vi "Cuboid collision and min distance test.vi"(2 "Cuboid 2":T1={"Vertices (x, y)"=[[0.0, 0.0], [0.0, 0.0], [0.0, 0.0], [0.0, 0.0]], "Zmin"=0.0, "Zmax"=0.0, "Centroid (x, y)"=[0.0, 0.0], "Radius"=0.0, "Edge normals (x, y)"=[[0.0, 0.0], [0.0, 0.0], [0.0, 0.0], [0.0, 0.0]], "Edge vectors (x, y)"=[[0.0, 0.0], [0.0, 0.0], [0.0, 0.0], [0.0, 0.0]]}, 3 "Cuboid 1":T1={"Vertices (x, y)"=[[0.0, 0.0], [0.0, 0.0], [0.0, 0.0], [0.0, 0.0]], "Zmin"=0.0, "Zmax"=0.0, "Centroid (x, y)"=[0.0, 0.0], "Radius"=0.0, "Edge normals (x, y)"=[[0.0, 0.0], [0.0, 0.0], [0.0, 0.0], [0.0, 0.0]], "Edge vectors (x, y)"=[[0.0, 0.0], [0.0, 0.0], [0.0, 0.0], [0.0, 0.0]]}) -> (0 "Minimum separation":dbl, 1 "Collision":bool)   [LabVIEW 2013]
uses:
  Cuboid properties.ctl
  <vilib>/Analysis/baseanly.llb/Real Dot Product.vi
  <vilib>/Analysis/NI_AALBase.lvlib
panel:
  # "PN 30/08/2014"
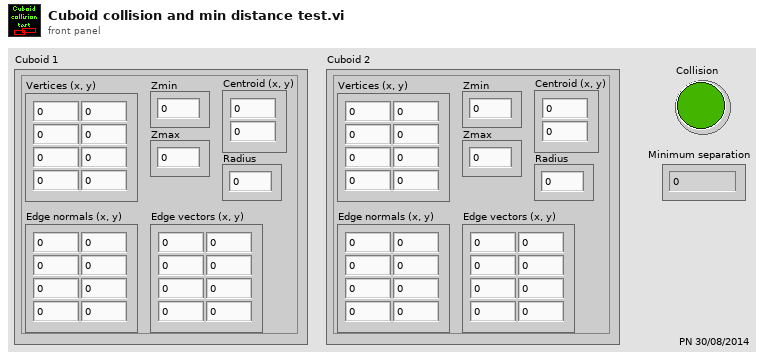
[diagram p1: front panel]
types:
  T1 = typedef "Cuboid properties.ctl" = cluster{"Vertices (x, y)":dbl[][], "Zmin":dbl, "Zmax":dbl, "Centroid (x, y)":dbl[], "Radius":dbl, "Edge normals (x, y)":dbl[][], "Edge vectors (x, y)":dbl[][]}
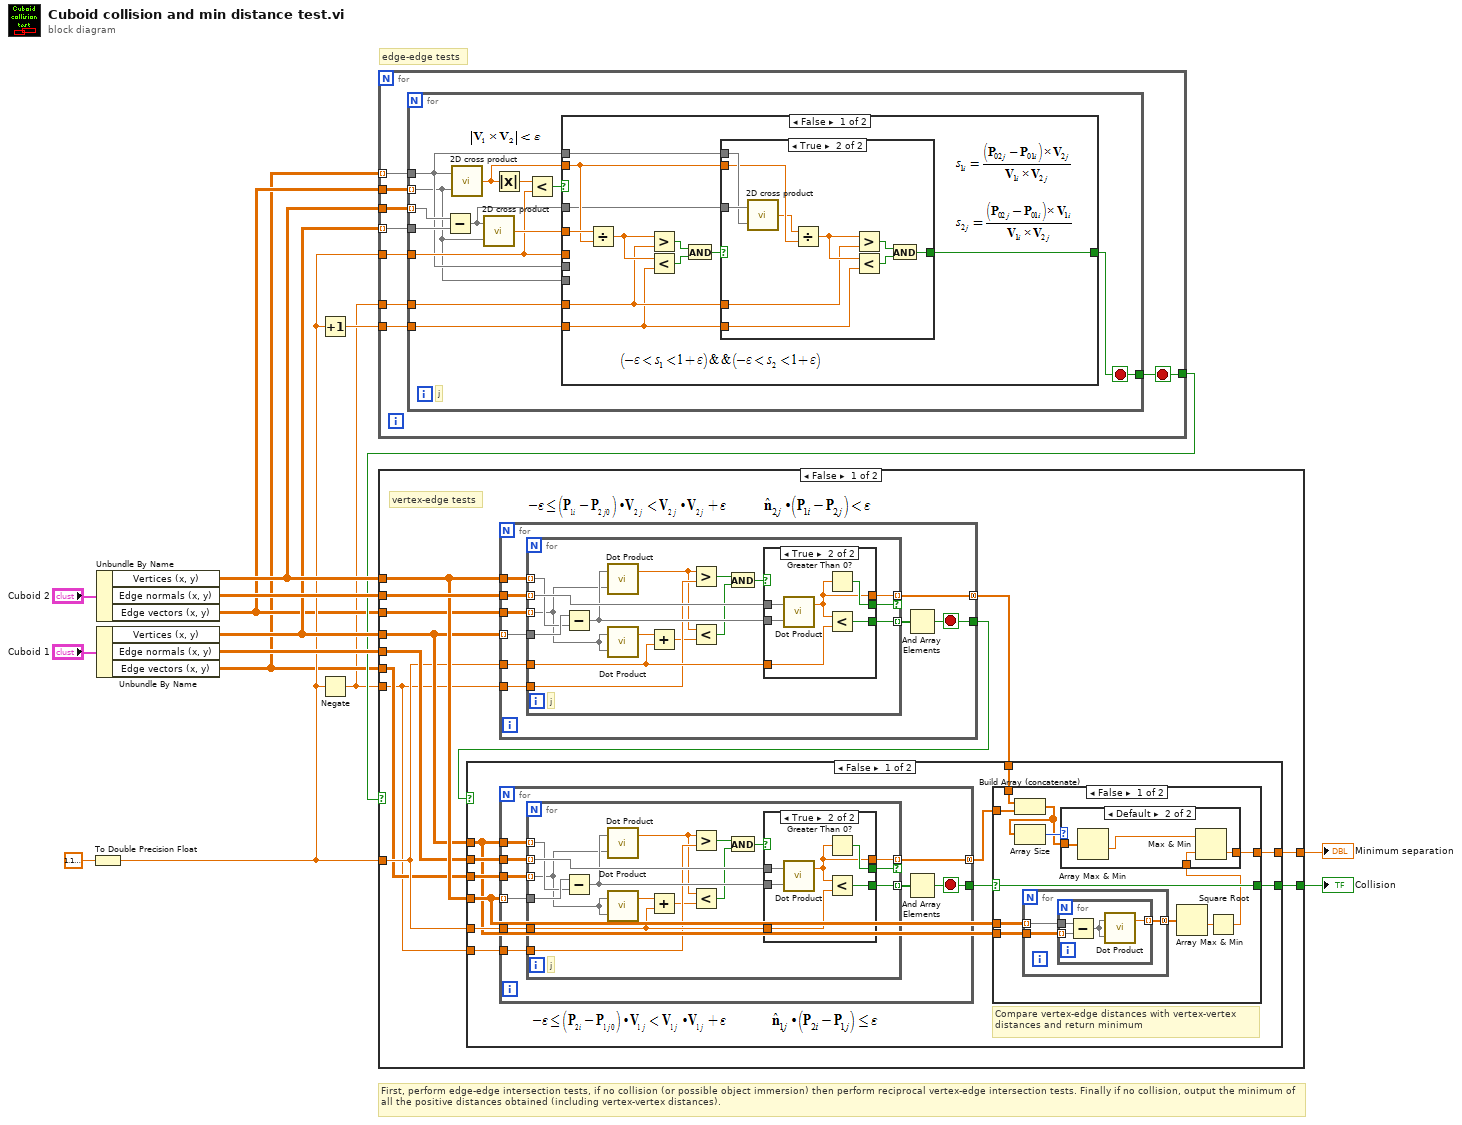
[diagram p0: block diagram]
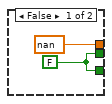
[diagram p2: hidden frame]
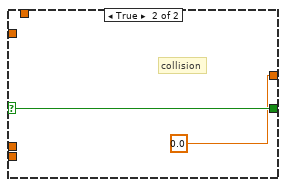
[diagram p4: hidden frame]
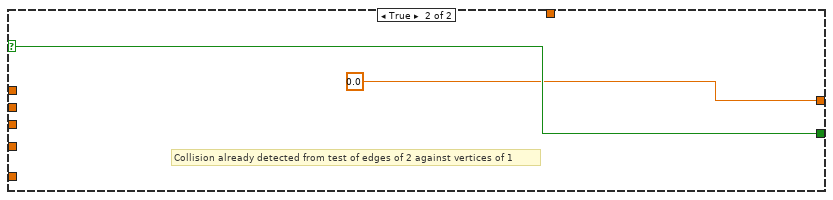
[diagram p5: hidden frame]
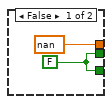
[diagram p6: hidden frame]
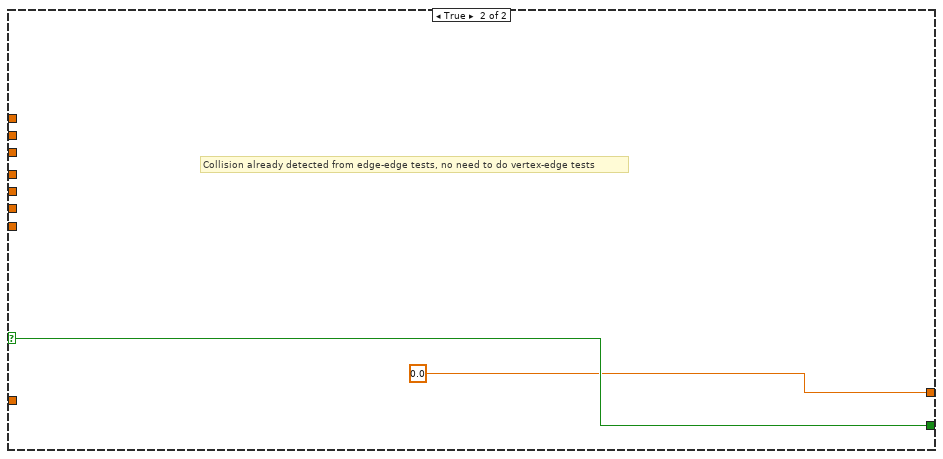
[diagram p7: hidden frame]
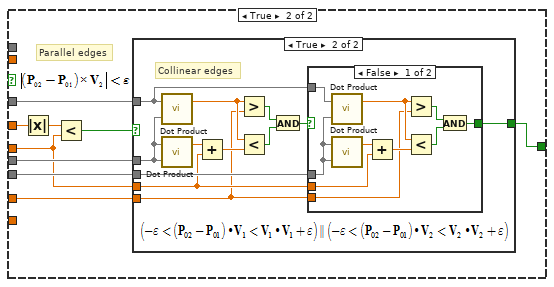
[diagram p9: hidden frame]
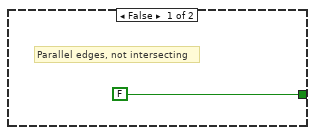
[diagram p10: hidden frame]
diagram:
  # "edge-edge tests"
  # "First, perform edge-edge intersection tests, if no collision (or possible object immersion) then perform reciprocal vertex-edge intersection tests. Finally if no collision, output the minimum of all the positive distances obtained (including vertex-vertex distances)."
  n1 = To Double Precision Float(number=sgl 1.1920929e-07) -> (double precision float=w5:dbl)
  n2 = Unbundle By Name("Cuboid 2") -> ("Vertices (x, y)"=w10:dbl[][], "Edge normals (x, y)"=w13:dbl[][], "Edge vectors (x, y)"=w3:dbl[][])
  n3 = Unbundle By Name("Cuboid 1") -> ("Vertices (x, y)"=w8:dbl[][], "Edge normals (x, y)"=w9:dbl[][], "Edge vectors (x, y)"=w2:dbl[][])
  n4 = Increment(x=w5) -> (x+1=w7:dbl)
  n5 = Negate(x=w5) -> (-x=w1:dbl)
  n6 = for {
    tunnel: w2 -> [w23] mode=indexing
    tunnel: w3 -> [w22]
    tunnel: w10 -> [w21]
    tunnel: w8 -> [w20] mode=indexing
    tunnel: w1 -> [w19]
    tunnel: w7 -> [w18]
    tunnel: w5 -> [w17]
    tunnel: [w16] -> w4
    stop <- w16 stop-if-true
    n7 = for {
      tunnel: w23 -> [w25]
      tunnel: w22 -> [w24] mode=indexing
      tunnel: w21 -> [w30] mode=indexing
      tunnel: w20 -> [w31]
      tunnel: w19 -> [w29]
      tunnel: w18 -> [w26]
      tunnel: w17 -> [w33]
      tunnel: [w28] -> w16
      stop <- w28 stop-if-true
      # "j"
      n8 = Subtract(x=w30, y=w31) -> (x-y=w32:dbl[])
      n9 = call "2D cross product.vi"("B"=w24, "A"=w25) -> ("A X B"=w27:dbl)
      n10 = call "2D cross product.vi"("B"=w24, "A"=w32) -> ("A X B"=w34:dbl)
      n11 = Absolute Value(x=w27) -> (abs(x)=w36:dbl)
      n12 = Less?(x=w36, y=w33) -> (x < y?=w35:bool)
      n13 = case shown="False" w35 {
        tunnel: w34 -> [w47 w67]
        tunnel: w33 -> [_ w60]
        tunnel: [w42 w64] -> w28
        tunnel: w32 -> [w40 w63]
        tunnel: w25 -> [_ w62]
        tunnel: w24 -> [_ w61]
        tunnel: w29 -> [w38 w59]
        tunnel: w27 -> [w41 _]
        tunnel: w26 -> [w37 _]
        tunnel: w25 -> [w39 _]
        frame False {
          n14 = Divide(x=w47, y=w41) -> (x/y=w46:dbl)
          n15 = Greater?(x=w46, y=w38) -> (0:w45:bool)
          n16 = Less?(x=w46, y=w37) -> (x < y?=w44:bool)
          n17 = And(x=w45, y=w44) -> (x .and. y?=w43:bool)
          n18 = case shown="True" w43 {
            selector: w43 -> [w48 _]
            tunnel: [w48 w51] -> w42
            tunnel: w41 -> [_ w53]
            tunnel: w40 -> [_ w55]
            tunnel: w39 -> [_ w54]
            tunnel: w38 -> [_ w50]
            tunnel: w37 -> [_ w49]
            frame False {
              # "not on edge"
            }
            frame True {
              n19 = call "2D cross product.vi"("B"=w54, "A"=w55) -> ("A X B"=w52:dbl)
              n20 = Divide(x=w52, y=w53) -> (x/y=w56:dbl)
              n21 = Greater?(x=w56, y=w50) -> (0:w57:bool)
              n22 = Less?(x=w56, y=w49) -> (x < y?=w58:bool)
              n23 = And(x=w57, y=w58) -> (x .and. y?=w51:bool)
            }
          }
        }
        frame True {
          # "Parallel edges"
          n24 = Absolute Value(x=w67) -> (abs(x)=w66:dbl)
          n25 = Less?(x=w66, y=w60) -> (x < y?=w65:bool)
          n26 = case shown="True" w65 {
            tunnel: [FALSE w73] -> w64
            tunnel: w63 -> [_ w72]
            tunnel: w62 -> [_ w80]
            tunnel: w61 -> [_ w71]
            tunnel: w60 -> [_ w70]
            tunnel: w59 -> [_ w69]
            frame False {
              # "Parallel edges, not intersecting"
            }
            frame True {
              # "Collinear edges"
              n27 = call-poly <vilib>:"Dot Product.vi"("Y Vector"=w80, "X Vector"=w72) -> ("X * Y"=w77:dbl)  [unwired: 1 out]
              n28 = call-poly <vilib>:"Dot Product.vi"("Y Vector"=w80, "X Vector"=w80) -> ("X * Y"=w79:dbl)  [unwired: 1 out]
              n29 = Add(x=w79, y=w70) -> (x+y=w78:dbl)
              n30 = Greater?(x=w77, y=w69) -> (0:w75:bool)
              n31 = Less?(x=w77, y=w78) -> (x < y?=w74:bool)
              n32 = And(x=w75, y=w74) -> (x .and. y?=w76:bool)
              n33 = case shown="False" w76 {
                selector: w76 -> [_ w91]
                tunnel: [w81 w91] -> w73
                tunnel: w72 -> [w90 _]
                tunnel: w71 -> [w89 _]
                tunnel: w70 -> [w87 _]
                tunnel: w69 -> [w82 _]
                frame False {
                  n34 = call-poly <vilib>:"Dot Product.vi"("Y Vector"=w89, "X Vector"=w90) -> ("X * Y"=w84:dbl)  [unwired: 1 out]
                  n35 = call-poly <vilib>:"Dot Product.vi"("Y Vector"=w89, "X Vector"=w89) -> ("X * Y"=w88:dbl)  [unwired: 1 out]
                  n36 = Add(x=w88, y=w87) -> (x+y=w83:dbl)
                  n37 = Greater?(x=w84, y=w82) -> (0:w85:bool)
                  n38 = Less?(x=w84, y=w83) -> (x < y?=w86:bool)
                  n39 = And(x=w85, y=w86) -> (x .and. y?=w81:bool)
                }
                frame True {
                  # "else disjoint"
                  # "overlapping"
                }
              }
            }
          }
        }
      }
    }
  }
  n40 = case shown="False" w4 {
    selector: w4 -> [_ w209]
    tunnel: w13 -> [w103 _]
    tunnel: [w101 w209] -> w12
    tunnel: [w100 0.0 ("tolerance (absolute)")] -> w11
    tunnel: w10 -> [w98 _]
    tunnel: w9 -> [w97 _]
    tunnel: w8 -> [w96 _]
    tunnel: w5 -> [w95 _]
    tunnel: w3 -> [w94 _]
    tunnel: w2 -> [w93 _]
    tunnel: w1 -> [w92 _]
    frame False {
      # "vertex-edge tests"
      n41 = for {
        tunnel: w103 -> [w183]
        tunnel: w96 -> [w182] mode=indexing
        tunnel: w98 -> [w181]
        tunnel: w95 -> [w180]
        tunnel: [w178] -> w102
        tunnel: w94 -> [w177]
        tunnel: w92 -> [w176]
        tunnel: [w175] -> w99 mode=concatenating
        stop <- w178 stop-if-true
        n42 = for {
          tunnel: [w193] -> w175 mode=indexing if=w196
          tunnel: w183 -> [w198] mode=indexing
          tunnel: w182 -> [w199]
          tunnel: w181 -> [w194] mode=indexing
          tunnel: w180 -> [w190]
          tunnel: [w197] -> w179 mode=indexing
          tunnel: w177 -> [w192] mode=indexing
          tunnel: w176 -> [w189]
          # "j"
          n43 = Subtract(x=w199, y=w194) -> (x-y=w195:dbl[])
          n44 = call-poly <vilib>:"Dot Product.vi"("Y Vector"=w192, "X Vector"=w195) -> ("X * Y"=w188:dbl)  [unwired: 1 out]
          n45 = call-poly <vilib>:"Dot Product.vi"("Y Vector"=w192, "X Vector"=w192) -> ("X * Y"=w191:dbl)  [unwired: 1 out]
          n46 = Add(x=w191, y=w190) -> (x+y=w187:dbl)
          n47 = Greater?(x=w188, y=w189) -> (0:w186:bool)
          n48 = Less?(x=w188, y=w187) -> (x < y?=w185:bool)
          n49 = And(x=w186, y=w185) -> (x .and. y?=w184:bool)
          n50 = case shown="True" w184 {
            tunnel: w198 -> [_ w207]
            tunnel: [w200 w206] -> w197
            tunnel: [w200 w205] -> w196
            tunnel: w195 -> [_ w204]
            tunnel: [nan ("X * Y") w203] -> w193
            tunnel: w190 -> [_ w202]
            frame False {
              w200 = FALSE
            }
            frame True {
              n51 = call-poly <vilib>:"Dot Product.vi"("Y Vector"=w204, "X Vector"=w207) -> ("X * Y"=w203:dbl)  [unwired: 1 out]
              n52 = Greater Than 0?(x=w203) -> (x > 0?=w205:bool)
              n53 = Less?(x=w203, y=w202) -> (x < y?=w206:bool)
            }
          }
        }
        n54 = And Array Elements(Boolean array=w179) -> (logical AND=w178:bool)
      }
      n55 = case shown="False" w102 {
        selector: w102 -> [_ w174]
        tunnel: [w114 w174] -> w101
        tunnel: [w113 0.0 ("tolerance (absolute)")] -> w100
        tunnel: w99 -> [w112 _]
        tunnel: w97 -> [w111 _]
        tunnel: w96 -> [w105 _]
        tunnel: w98 -> [w106 _]
        tunnel: w95 -> [w109 _]
        tunnel: w93 -> [w110 _]
        tunnel: w92 -> [w108 _]
        frame False {
          # "Compare vertex-edge distances with vertex-vertex distances and return minimum"
          n56 = for {
            tunnel: w111 -> [w123]
            tunnel: w106 -> [w122] mode=indexing
            tunnel: w105 -> [w121]
            tunnel: w109 -> [w120]
            tunnel: [w118] -> w107
            tunnel: w110 -> [w117]
            tunnel: w108 -> [w116]
            tunnel: [w115] -> w104 mode=concatenating
            stop <- w118 stop-if-true
            n57 = for {
              tunnel: [w133] -> w115 mode=indexing if=w136
              tunnel: w123 -> [w138] mode=indexing
              tunnel: w122 -> [w139]
              tunnel: w121 -> [w134] mode=indexing
              tunnel: w120 -> [w130]
              tunnel: [w137] -> w119 mode=indexing
              tunnel: w117 -> [w132] mode=indexing
              tunnel: w116 -> [w129]
              # "j"
              n58 = Subtract(x=w139, y=w134) -> (x-y=w135:dbl[])
              n59 = call-poly <vilib>:"Dot Product.vi"("Y Vector"=w132, "X Vector"=w135) -> ("X * Y"=w128:dbl)  [unwired: 1 out]
              n60 = call-poly <vilib>:"Dot Product.vi"("Y Vector"=w132, "X Vector"=w132) -> ("X * Y"=w131:dbl)  [unwired: 1 out]
              n61 = Add(x=w131, y=w130) -> (x+y=w127:dbl)
              n62 = Greater?(x=w128, y=w129) -> (0:w126:bool)
              n63 = Less?(x=w128, y=w127) -> (x < y?=w125:bool)
              n64 = And(x=w126, y=w125) -> (x .and. y?=w124:bool)
              n65 = case shown="True" w124 {
                tunnel: w138 -> [_ w147]
                tunnel: [w140 w146] -> w137
                tunnel: [w140 w145] -> w136
                tunnel: w135 -> [_ w144]
                tunnel: [nan ("X * Y") w143] -> w133
                tunnel: w130 -> [_ w142]
                frame False {
                  w140 = FALSE
                }
                frame True {
                  n66 = call-poly <vilib>:"Dot Product.vi"("Y Vector"=w144, "X Vector"=w147) -> ("X * Y"=w143:dbl)  [unwired: 1 out]
                  n67 = Greater Than 0?(x=w143) -> (x > 0?=w145:bool)
                  n68 = Less?(x=w143, y=w142) -> (x < y?=w146:bool)
                }
              }
            }
            n69 = And Array Elements(Boolean array=w119) -> (logical AND=w118:bool)
          }
          n70 = case shown="False" w107 {
            selector: w107 -> [w154 w172]
            tunnel: [w154 w172] -> w114
            tunnel: [w148 0.0 ("tolerance (absolute)")] -> w113
            tunnel: w112 -> [w158 _]
            tunnel: w104 -> [w157 _]
            tunnel: w106 -> [w150 _]
            tunnel: w105 -> [w151 _]
            frame False {
              n71 = Build Array (concatenate)(w158, w157) -> (w155:dbl[])
              n72 = Array Size(array=w155) -> (size(s)=w156:i32)
              n73 = for {
                tunnel: [w161] -> w152 mode=concatenating
                tunnel: w150 -> [w160] mode=indexing
                tunnel: w151 -> [w159]
                n74 = for {
                  tunnel: [w164] -> w161 mode=indexing
                  tunnel: w160 -> [w163]
                  tunnel: w159 -> [w162] mode=indexing
                  n75 = Subtract(x=w163, y=w162) -> (x-y=w165:dbl[])
                  n76 = call-poly <vilib>:"Dot Product.vi"("Y Vector"=w165, "X Vector"=w165) -> ("X * Y"=w164:dbl)  [unwired: 1 out]
                }
              }
              n77 = Array Max & Min(array=w152) -> (min value=w153:dbl)  [unwired: 3 out]
              n78 = Square Root(x=w153) -> (sqrt(x)=w149:dbl)
              n79 = case shown="Default" w156 {
                tunnel: w155 -> [_ w170]
                tunnel: [w166 w167] -> w148
                tunnel: w149 -> [w166 w169]
                frame 0 {
                }
                frame Default {
                  n80 = Array Max & Min(array=w170) -> (min value=w168:dbl)  [unwired: 3 out]
                  n81 = Max & Min(x=w168, y=w169) -> (min(x,y)=w167:dbl)  [unwired: 1 out]
                }
              }
            }
            frame True {
              # "collision"
            }
          }
        }
        frame True {
          # "Collision already detected from test of edges of 2 against vertices of 1"
        }
      }
    }
    frame True {
      # "Collision already detected from edge-edge tests, no need to do vertex-edge tests"
    }
  }
  "Collision" <- w12
  "Minimum separation" <- w11
